vi "ReadResponse.vi"(8 "error in (no error)":errorcluster, 11 "Port":refnum<visa-resource-name>) -> (0 "error out":errorcluster, 2 "Response":string, 3 "Port Out":refnum<visa-resource-name>)   [LabVIEW 2018]
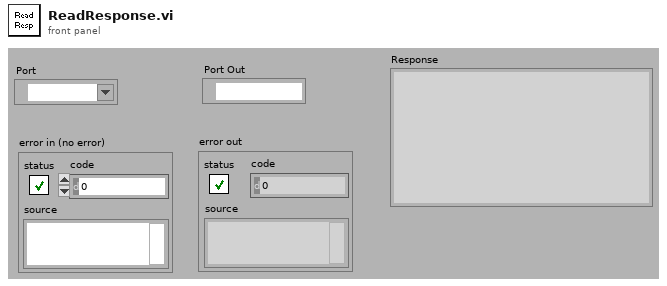
[diagram p1: front panel]
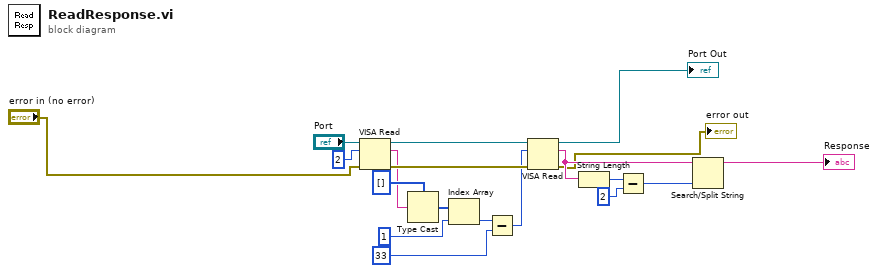
[diagram p0: block diagram]
diagram:
  n1 = VISA Read(VISA resource name="Port", byte count=u32 2, error in (no error)="error in (no error)") -> (VISA resource name out=w16:refnum<visa-resource-name>, read buffer=w10:string, error out=w18:errorcluster)  [unwired: 1 out]
  n2 = Type Cast(type=u8[] [], x=w10) -> (*(type *) &x=w12:u8[])
  n3 = Index Array(array=w12, index=1) -> (element=w14:u8)
  n4 = Subtract(x=w14, y=u8 33) -> (x-y=w17:u8)
  n5 = VISA Read(VISA resource name=w16, byte count=w17, error in (no error)=w18) -> (VISA resource name out=→"Port Out":refnum<visa-resource-name>, read buffer=w7:string, error out=→"error out":errorcluster)  [unwired: 1 out]
  n6 = String Length(string=w7) -> (length=w6:i32)
  n7 = Subtract(x=w6, y=2 ("x")) -> (x-y=w5:i32)
  n8 = Search/Split String(string=w7, offset (0)=w5) -> (substring before match=→"Response":string)  [unwired: 1 in, 2 out]
